vi "GetType.vi"(8 "error in (no error)":errorcluster, 11 "Configure Arb Frequency [AF] Msg":refnum<class "Configure Arb Frequency [AF] Msg.lvclass">) -> (0 "error out":errorcluster, 2 "Data Sample":variant, 3 "Configure Arb Frequency [AF] Msg":refnum<class "Configure Arb Frequency [AF] Msg.lvclass">)   [LabVIEW 2016, in "CS++Fgen.lvlib" / "Configure Arb Frequency [AF] Msg.lvclass"]
doc: "This VI delivers a sample of the data type format the message expects."
uses:
  Configure Arb Frequency [AF] Msg.lvclass
  Configure Arb Frequency [AF] Msg.lvclass/Configure Arb Frequency [AF] Msg.ctl
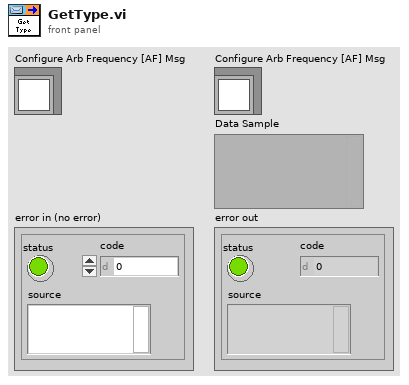
[diagram p1: front panel]
types:
  T1 = cluster{"channel name (\"CHANNEL1\")":string, "frequency (0.0 Hz)":dbl[unit]}
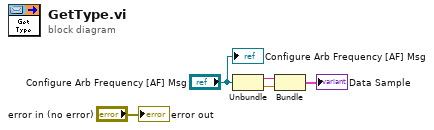
[diagram p0: block diagram]
diagram:
  n1 = Unbundle("Configure Arb Frequency [AF] Msg") -> (w2:string, w1:dbl[unit])
  n2 = Bundle("channel name (\"CHANNEL1\")"=w2, "frequency (0.0 Hz)"=w1) -> (→"Data Sample":T1)  [unwired: 1 in]
  "error out" <- "error in (no error)"
  "Configure Arb Frequency [AF] Msg" <- "Configure Arb Frequency [AF] Msg"
